vi "Klinger UpdateByRef.vi"(0 "Moving?":bool, 5 "Moving Ref":refnum<vi>, 7 "Position":dbl, 9 "Position Ref":refnum<vi>, 11 "error in":errorcluster) -> (15 "error out":errorcluster)   [LabVIEW 2010]
doc: "Ce VI rafraîchit l'affichage des contrôles dont les références lui sont connectées. Il permet l'affichage en temps réel de la position et du statut \"mouvement en cours\"."
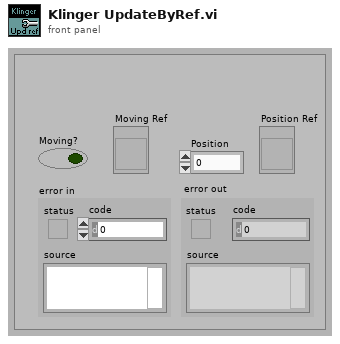
[diagram p1: front panel]
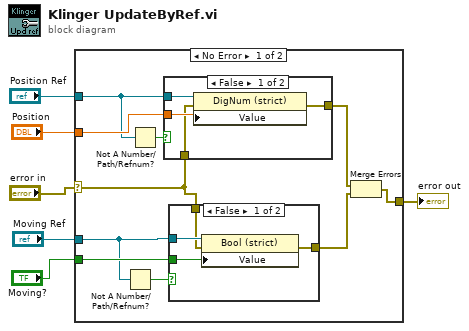
[diagram p0: block diagram]
diagram:
  n1 = case shown="No Error" "error in" {
    selector: "error in" -> [w7 w27]
    tunnel: "Position" -> [w16 _]
    tunnel: "Moving?" -> [w15 _]
    tunnel: "Position Ref" -> [w12 _]
    tunnel: "Moving Ref" -> [w11 _]
    tunnel: [w8 w27] -> w2
    frame No Error {
      n2 = Not A Number/Path/Refnum?(number/path/refnum=w11) -> (NaN/Path/Refnum?=w14:bool)
      n3 = Not A Number/Path/Refnum?(number/path/refnum=w12) -> (NaN/Path/Refnum?=w13:bool)
      n4 = case shown="False" w13 {
        tunnel: w16 -> [w25 _]
        tunnel: w12 -> [w24 _]
        tunnel: w7 -> [w23 w26]
        tunnel: [w22 w26] -> w10
        frame False {
          n5 = property class="DigNum (strict)"(reference=w24, error in=w23, "Value"=w25) -> (error out=w22:errorcluster)  [unwired: 1 out]
        }
        frame True {
        }
      }
      n6 = case shown="False" w14 {
        tunnel: w11 -> [w20 _]
        tunnel: w15 -> [w19 _]
        tunnel: w7 -> [w18 w21]
        tunnel: [w17 w21] -> w9
        frame False {
          n7 = property class="Bool (strict)"(reference=w20, error in=w18, "Value"=w19) -> (error out=w17:errorcluster)  [unwired: 1 out]
        }
        frame True {
        }
      }
      n8 = Merge Errors(w10, w9) -> (w8:errorcluster)
    }
    frame Error {
    }
  }
  "error out" <- w2
